vi "Sturms Chain Single Roots.vi"(11 "f":dbl[](array[numeric])) -> (3 "sequence of polynomials":dbl[][](array[numeric]))   [LabVIEW 2018, in "NI_AALPro.lvlib"]
doc: "From ../labview/vi.lib/gmath/zeros.llb."
uses:
  <vilib>/Analysis/NI_AALPro.lvlib
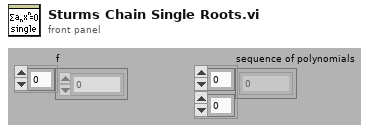
[diagram p1: front panel]
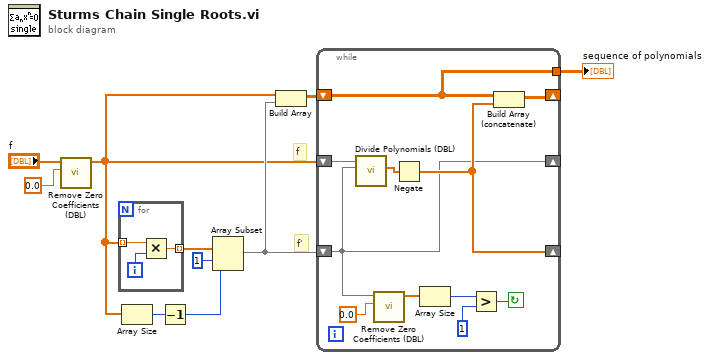
[diagram p0: block diagram]
diagram:
  # "f'"
  # "f"
  n1 = call "Remove Zero Coefficients (DBL).vi"("threshold"=0.0, "P(x) In"="f") -> ("P(x) Out"=w5:dbl[])  [unwired: 7 in, 2 out]
  n2 = for {
    tunnel: w5 -> [w13] mode=indexing
    tunnel: [w11] -> w10 mode=indexing
    i -> [w12]
    n3 = Multiply(x=w13, y=w12) -> (x*y=w11:dbl)
  }
  n4 = Array Size(array=w5) -> (size(s)=w7:i32)
  n5 = Decrement(x=w7) -> (x-1=w9:i32)
  n6 = Array Subset(array=w10, index=1, length=w9) -> (w6:dbl[])
  n7 = Build Array(w5, w6) -> (w4:dbl[][])
  n8 = while {
    tunnel: [w17] -> w2
    shift-left: w6 -> [w16]
    shift-right: [w23] -> _
    shift-left: w5 -> [w21]
    shift-right: [w16] -> _
    shift-left: w4 -> [w17]
    shift-right: [w22] -> _
    stop <- w18 continue-if-true
    n9 = call "Divide Polynomials (DBL).vi"("Q(x)"=w16, "P(x)"=w21) -> ("Remainder"=w24:dbl[])  [unwired: 7 in, 2 out]
    n10 = call "Remove Zero Coefficients (DBL).vi"("threshold"=0.0, "P(x) In"=w16) -> ("P(x) Out"=w15:dbl[])  [unwired: 7 in, 2 out]
    n11 = Negate(x=w24) -> (-x=w23:dbl[])
    n12 = Array Size(array=w15) -> (size(s)=w20:i32)
    n13 = Greater?(x=w20, y=1) -> (0:w18:bool)
    n14 = Build Array (concatenate)(w17, w23) -> (w22:dbl[][])
  }
  "sequence of polynomials" <- w2
